vi "ADIS16448 Loop.vi"(8 "error in":errorcluster) -> ()   [LabVIEW 2019]
uses:
  Typedef/ADIS16448 Device Reference.ctl
  Typedef/ADIS16448 Hardware Configuration.ctl
  <vilib>/Rock Robotics/WPI/SPI/WPI_SPIMode.ctl
  <vilib>/Rock Robotics/SystemInterfaces/DIO/FPGA_DIOChannel.ctl
  <vilib>/Rock Robotics/SystemInterfaces/spilib/spi_bus.ctl
  Typedef/ADIS16448 Status.ctl
  Typedef/ADIS16448 Data.ctl
  Typedef/ADIS16448 Process.ctl
  Typedef/ADIS16448 Command Type.ctl
  <vilib>/Rock Robotics/SystemInterfaces/CounterEncoderSourceConvertion/FPGA_CounterEncoderSourceConvertionLVSourceType.ctl
  <vilib>/Rock Robotics/SystemInterfaces/DIO/FPGA_DIODigitalSourceChannel.ctl
  <vilib>/Rock Robotics/SystemInterfaces/AnalogTrigger/FPGA_AnalogTriggerIndex.ctl
  <vilib>/Rock Robotics/SystemInterfaces/AnalogTrigger/FPGA_AnalogTriggerOutType.ctl
  <vilib>/Rock Robotics/WPI/SPI/WPI_SPIDevRef.ctl
  Typedef/ADIS16448 Register.ctl
  <vilib>/Rock Robotics/WPI/Counter/WPI_CounterDigitalInputToDigitalSource.vi
  <vilib>/ptbypt/NI_PtbyPt.lvlib
panel:
  in  "Calibration Time":i32
  in  "element":T1
  in  "ADIS16448DevRef":T2={"DevStatus"={"status"=FALSE, "code"=0, "source"=""}, "Hardware Config"={"SPI Clock Rate (Hz)"=1000000.0, "IMU SPI Mode (3)"=enum."Mode 3 (Clk Idle High,Sample on Trailing)", "IMU Reset Pin"=enum."SPI Port CS2", "IMU SPI Bus"=enum."SPI On-Board, CS0", "IMU Data Ready Pin"=enum."SPI Port CS1", "Stall Config"={"Pow2BytesPerRead"=255, "StallTicks"=640, "CsToSclkTicks"=5}, "IMU Status LED Pin"=enum."DIO MXP 9"}, "Calibration Complete"=refnum, "Status FIFO"=refnum, "Last Value Reference"=refnum, "Sychronous Process VI"=refnum, "Cmd FIFO"=refnum, "Source"={"DevStatus"={"status"=FALSE, "code"=0, "source"=""}, "AnalogTriggerMode?"=FALSE, "DigitalMode"={"DIO Channel"=enum."Disabled"}, "AnalogTriggerMode"={"AnalogTriggerIndex"=enum."Trig 0", "OutputType"=enum."InWindow"}}, "Data FIFO"=refnum, "IMU Status LED Pin"=enum."DIO MXP 9", "Calibration Time"=5}
  in  "Main Name":string
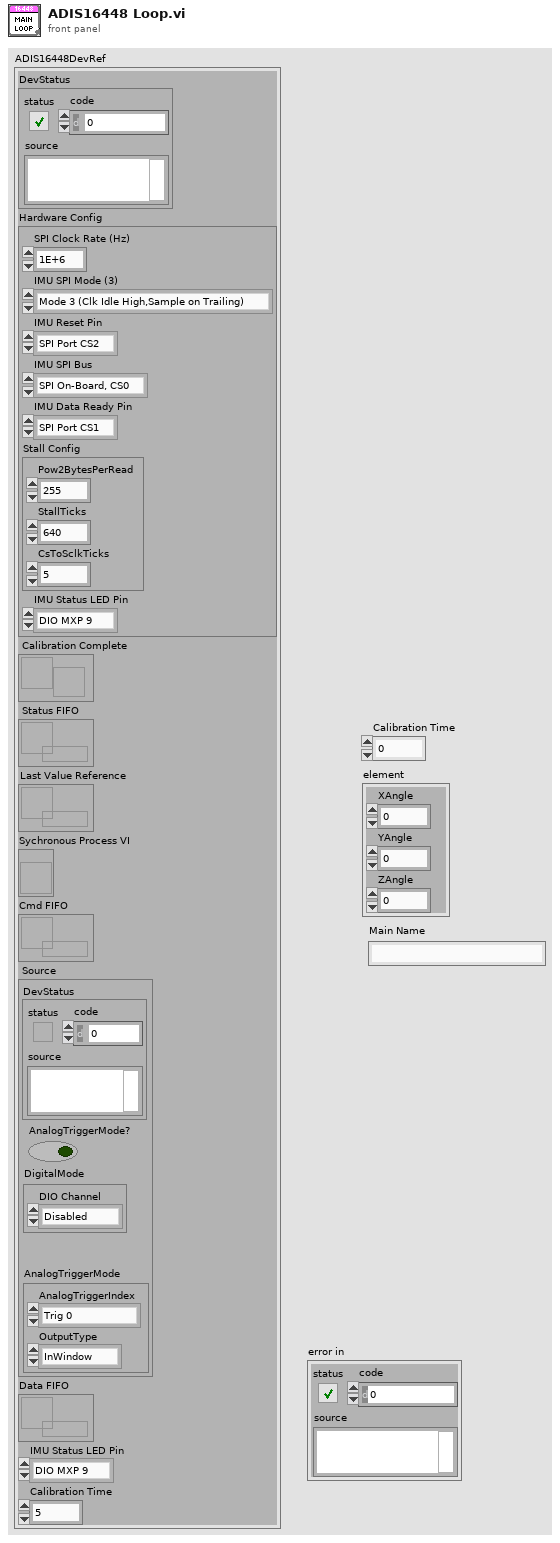
[diagram p1: front panel]
types:
  T1 = typedef "ADIS16448 Data.ctl" = cluster{"XAngle":dbl, "YAngle":dbl, "ZAngle":dbl}
  T2 = typedef "ADIS16448 Device Reference.ctl" = cluster{"DevStatus":errorcluster, "Hardware Config":T3, "Calibration Complete":refnum<notifier>, "Status FIFO":refnum<k33>, "Last Value Reference":refnum<data-value>, "Sychronous Process VI":T7, "Cmd FIFO":refnum<k33>, "Source":T8, "Data FIFO":refnum<k33>, "IMU Status LED Pin":T5, "Calibration Time":u32}
  T3 = typedef "ADIS16448 Hardware Configuration.ctl" = cluster{"SPI Clock Rate (Hz)":dbl, "IMU SPI Mode (3)":T4, "IMU Reset Pin":T5, "IMU SPI Bus":T6, "IMU Data Ready Pin":T5, "Stall Config":cluster{"Pow2BytesPerRead":u8, "StallTicks":u16, "CsToSclkTicks":u8}, "IMU Status LED Pin":T5}
  T4 = typedef "WPI_SPIMode.ctl" = enum16{"Mode 0 (Clk Idle Low,Sample on Leading)", "Mode 1 (Clk Idle Low,Sample on Trailing)", "Mode 2 (Clk Idle High,Sample on Leading)", "Mode 3 (Clk Idle High,Sample on Trailing)"}
  T5 = typedef "FPGA_DIOChannel.ctl" = enum8{"DIO 0", "DIO 1", "DIO 2", "DIO 3", "DIO 4", "DIO 5", "DIO 6", "DIO 7", "DIO 8", "DIO 9", "DIO MXP 0", "DIO MXP 1", "DIO MXP 2", "DIO MXP 3", "DIO MXP 4", "DIO MXP 5", "DIO MXP 6", "DIO MXP 7", "DIO MXP 8", "DIO MXP 9", "DIO MXP 10", "DIO MXP 11", "DIO MXP 12", "DIO MXP 13", "DIO MXP 14", "DIO MXP 15", "SPI Port CS1", "SPI Port CS2", "SPI Port CS3", "SPI Port MISO", "SPI Port MOSI", "Invalid"}
  T6 = typedef "spi_bus.ctl" = enum16{"SPI On-Board, CS0", "SPI On-Board, CS1", "SPI On-Board, CS2", "SPI On-Board, CS3", "SPI MXP", "Invalid"}
  T7 = typedef "ADIS16448 Process.ctl" = refnum<vi>
  T8 = typedef "FPGA_CounterEncoderSourceConvertionLVSourceType.ctl" = cluster{"DevStatus":errorcluster, "AnalogTriggerMode?":bool, "DigitalMode":cluster{"DIO Channel":T9}, "AnalogTriggerMode":cluster{"AnalogTriggerIndex":T10, "OutputType":T11}}
  T9 = typedef "FPGA_DIODigitalSourceChannel.ctl" = enum8{"DIO 0", "DIO 1", "DIO 2", "DIO 3", "DIO 4", "DIO 5", "DIO 6", "DIO 7", "DIO 8", "DIO 9", "DIO MXP 0", "DIO MXP 1", "DIO MXP 2", "DIO MXP 3", "DIO MXP 4", "DIO MXP 5", "DIO MXP 6", "DIO MXP 7", "DIO MXP 8", "DIO MXP 9", "DIO MXP 10", "DIO MXP 11", "DIO MXP 12", "DIO MXP 13", "DIO MXP 14", "DIO MXP 15", "SPI Port CS1", "SPI Port CS2", "SPI Port CS3", "SPI Port MISO", "SPI Port MOSI", "Disabled"}
  T10 = typedef "FPGA_AnalogTriggerIndex.ctl" = enum8{"Trig 0", "Trig 1", "Trig 2", "Trig 3", "Trig 4", "Trig 5", "Trig 6", "Trig 7", "Invalid"}
  T11 = typedef "FPGA_AnalogTriggerOutType.ctl" = enum16{"InWindow", "TriggerState", "Rising", "Falling"}
  T12 = typedef "WPI_SPIDevRef.ctl" = cluster{"DevStatus":errorcluster, "Handle":i32, "SPI Bus":T6}
  T13 = cluster{"SPIDevRef":T12, "Data Counter":u16, "Reset":bool, "Digital Source":T8, "Bytes Per Sample":u32, "Data":dbl[], "ADIS16448DevRef":T2, "TimeStampPrev":u32, "Sensor to Robot Rotation":dbl[][], "AutoSPI Active?":bool, "Offsets":dbl[], "Offset Counter":i32, "Data Header":u8[], "Zero Byte Count":u8, "Running Offset":dbl[]}
  T14 = typedef "ADIS16448 Status.ctl" = cluster{"Calibrated?":bool, "IMU Detected?":bool}
  T15 = typedef "ADIS16448 Register.ctl" = u8
  T16 = typedef "ADIS16448 Command Type.ctl" = cluster{"Command":enum16{"None", "Reset", "Rewrite Config", "Start Recal", "Recalibrate", "Recal Complete", "Exit Auto SPI", "Start Auto SPI", "Configure Cal"}, "Data":u32}
  T17 = typedef "WPI_DigitalOutputDevRef.ctl" = cluster{"DIO Channel":T5, "DevStatus":errorcluster}
  T18 = typedef "WPI_DigitalInputDevRef.ctl" = cluster{"DevStatus":errorcluster, "DIO Channel":T5}
  T19 = cluster{"Pow2BytesPerRead":u8, "StallTicks":u16, "CsToSclkTicks":u8}
  T20 = enum16{"None", "Reset", "Rewrite Config", "Start Recal", "Recalibrate", "Recal Complete", "Exit Auto SPI", "Start Auto SPI", "Configure Cal"}
  T21 = enum32{"Bad", "Idle", "Run top level", "Running"}
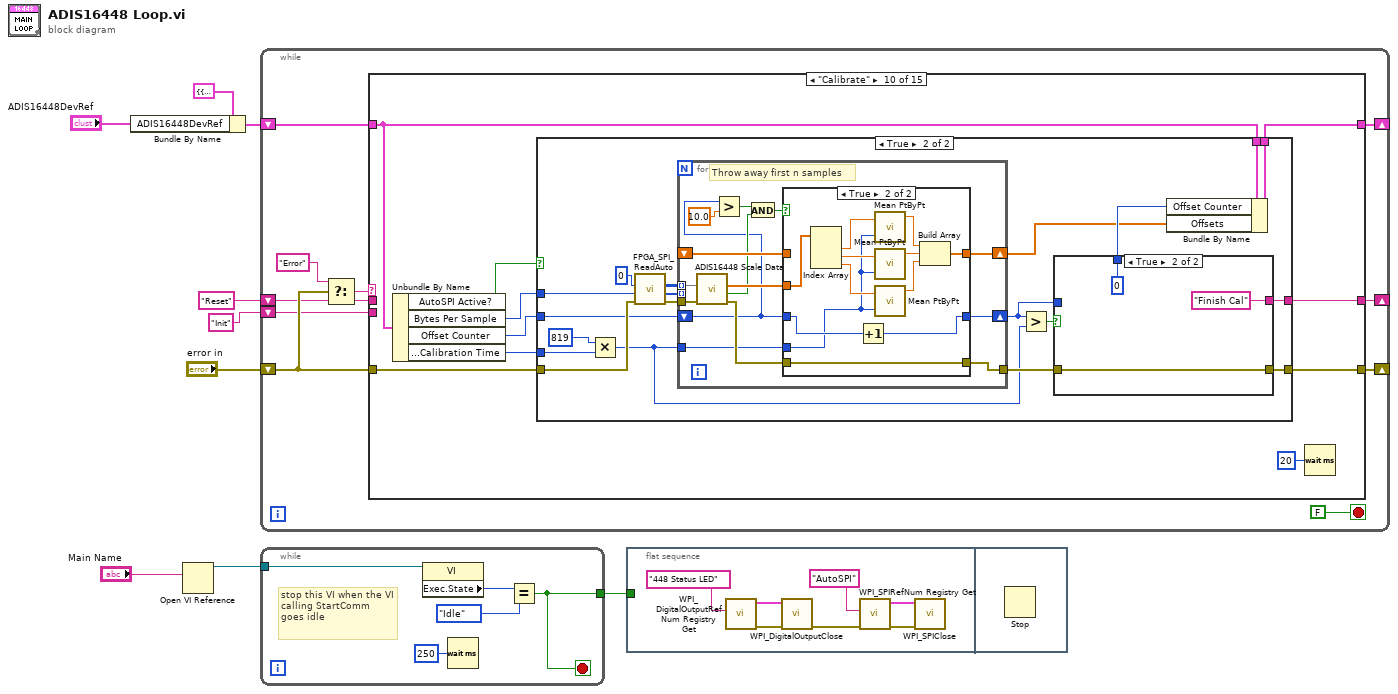
[diagram p0: block diagram]
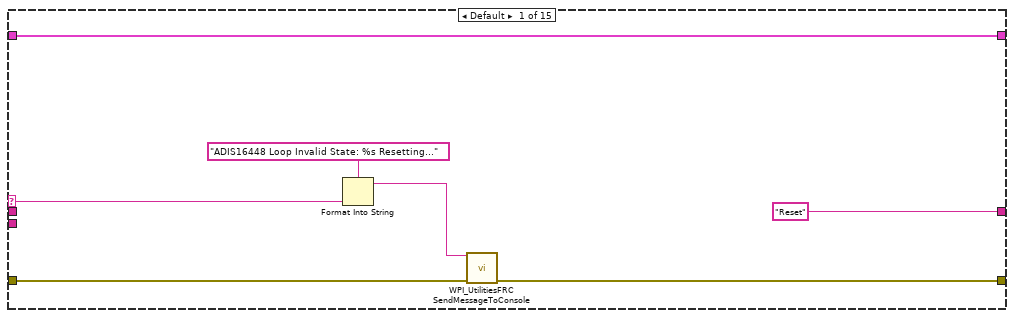
[diagram p2: hidden frame]
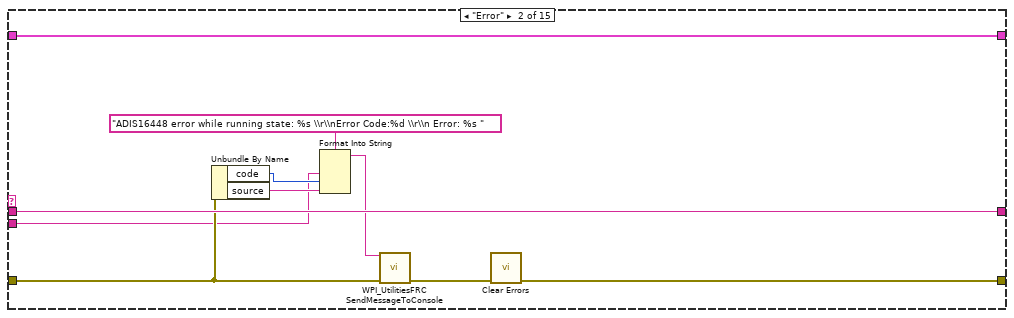
[diagram p3: hidden frame]
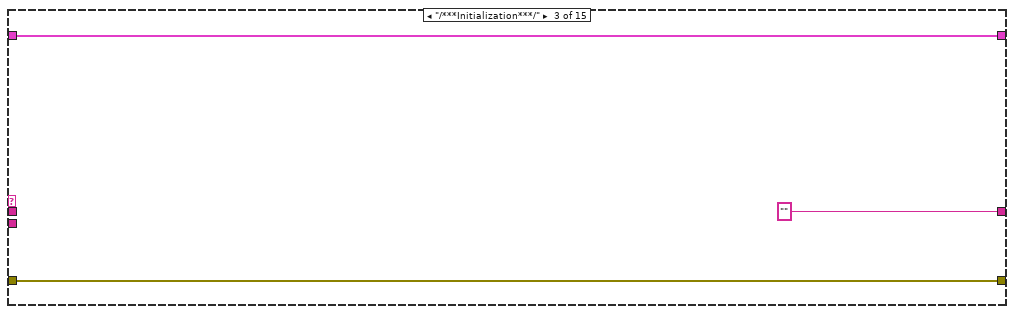
[diagram p4: hidden frame]
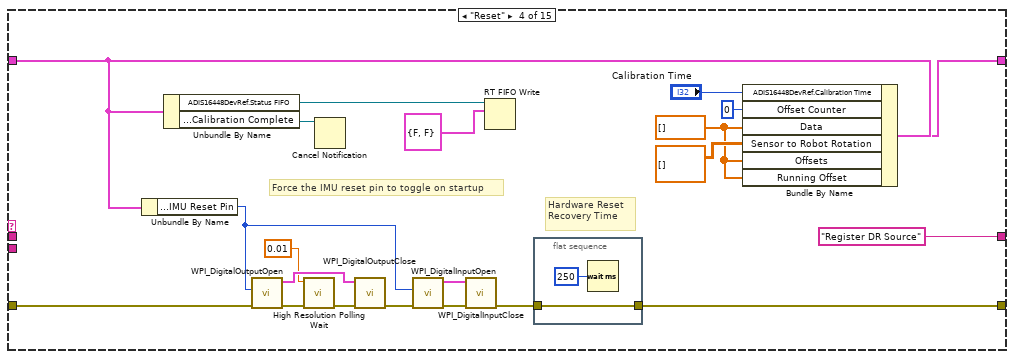
[diagram p5: hidden frame]
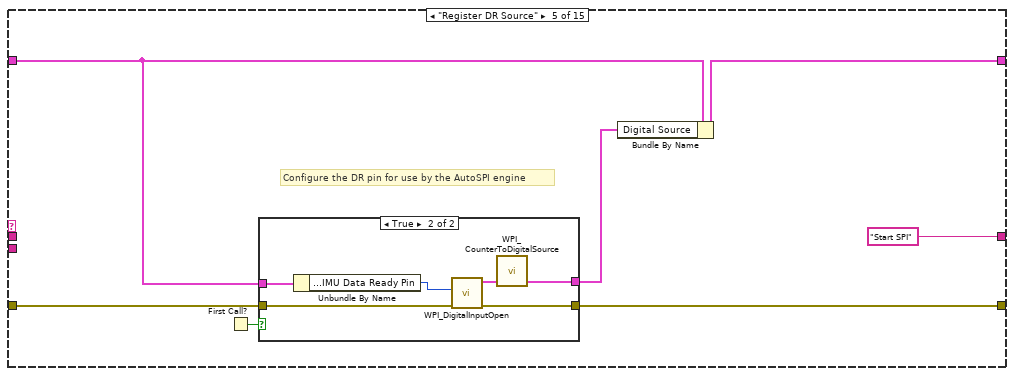
[diagram p6: hidden frame]
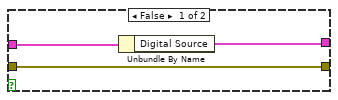
[diagram p7: hidden frame]
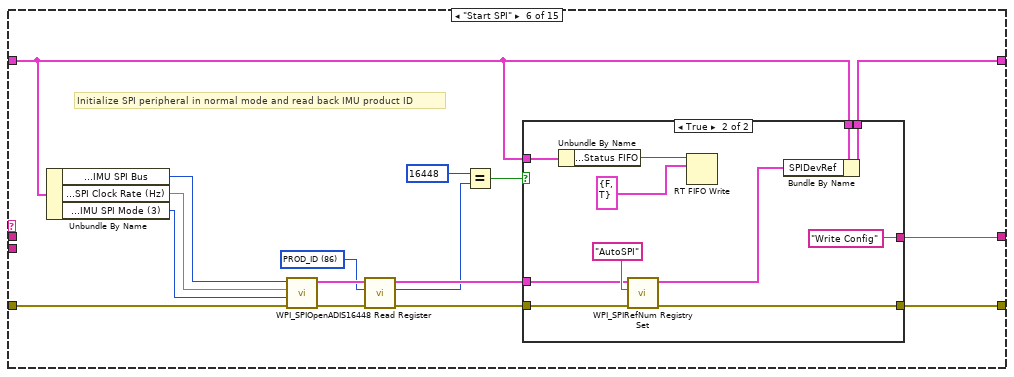
[diagram p8: hidden frame]
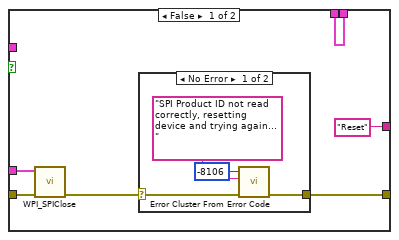
[diagram p9: hidden frame]
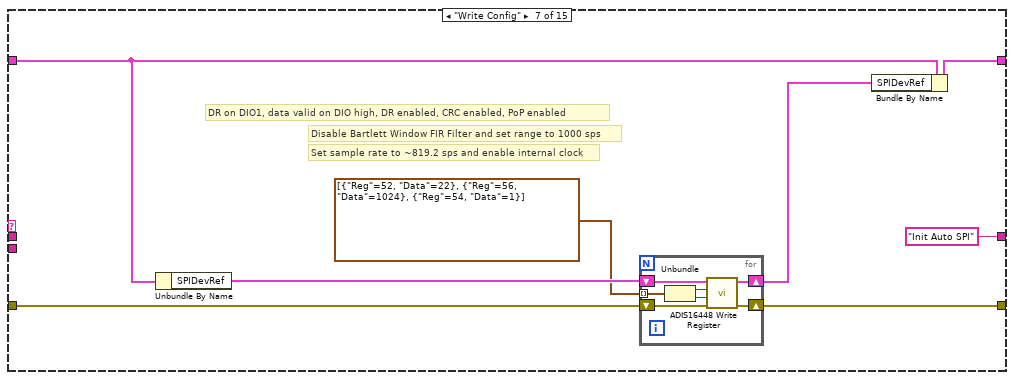
[diagram p11: hidden frame]
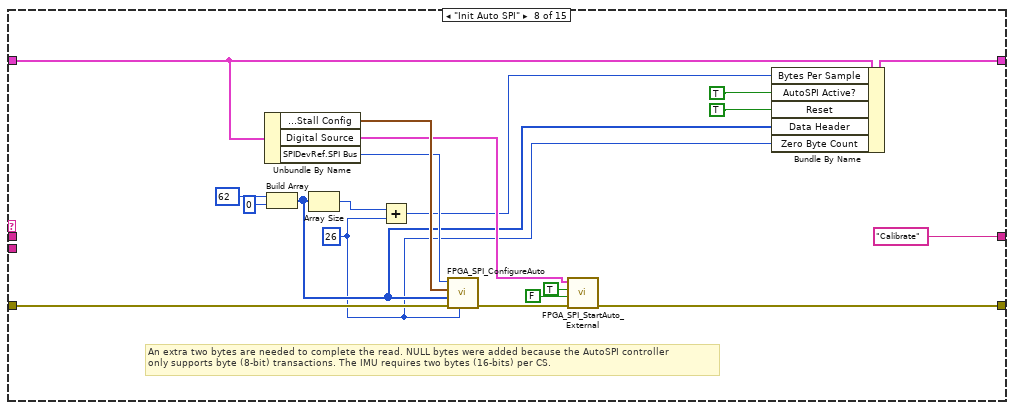
[diagram p12: hidden frame]
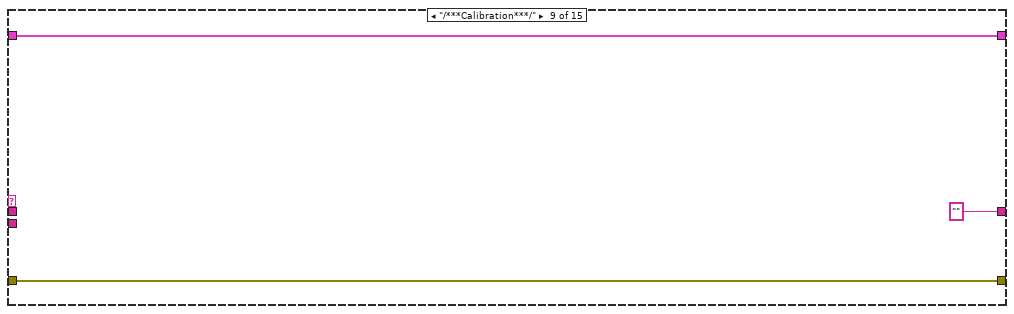
[diagram p13: hidden frame]
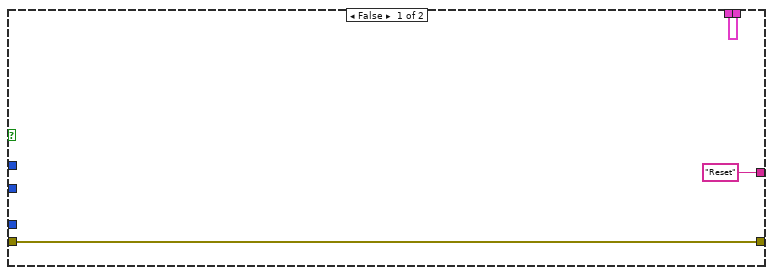
[diagram p14: hidden frame]
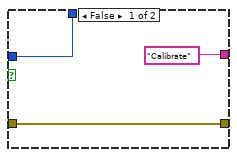
[diagram p15: hidden frame]
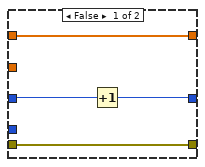
[diagram p16: hidden frame]
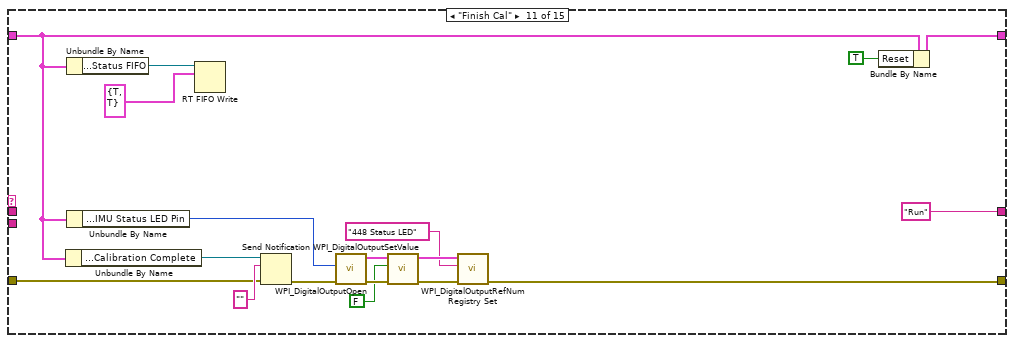
[diagram p17: hidden frame]
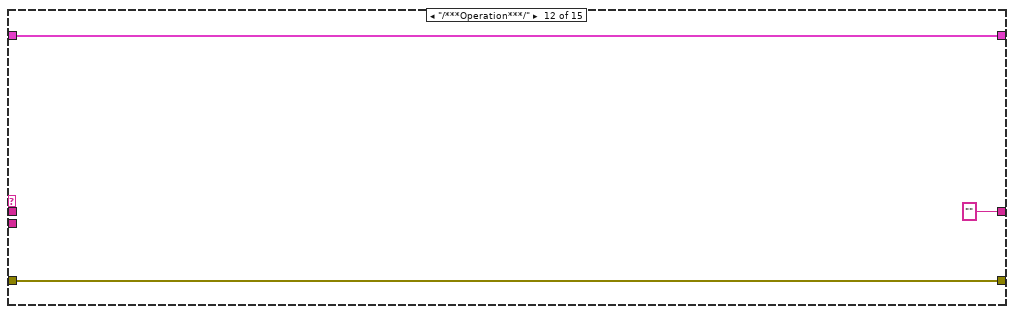
[diagram p18: hidden frame]
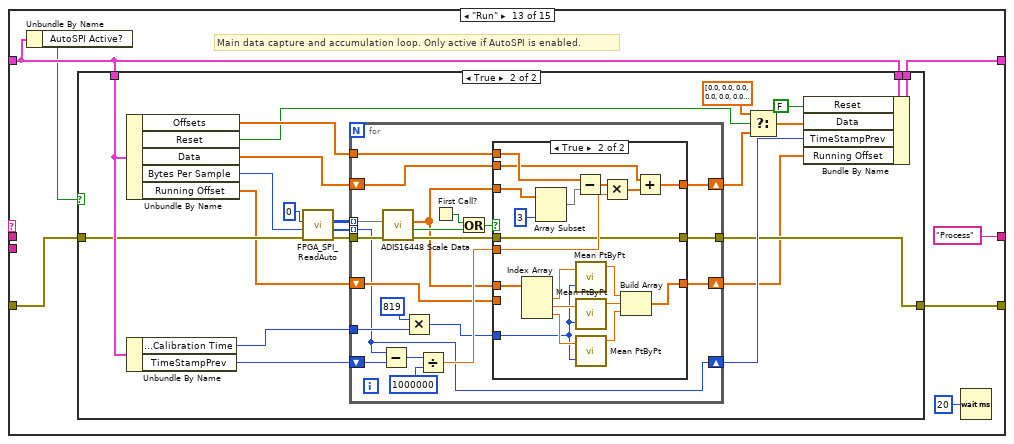
[diagram p19: hidden frame]
diagram:
  n1 = Bundle By Name(cluster=T13 {"SPIDevRef"={"DevStatus"={"status"=FALSE, "code"=0, "source"=""}, "Handle"=0, "SPI Bus"=enum."SPI On-Board, CS0"}, "Data Counter"=0, "Reset"=FALSE, "Digital Source"={"DevStatus"={"status"=FALSE, "code"=0, "source"=""}, "AnalogTriggerMode?"=FALSE, "DigitalMode"={"DIO Channel"=enum."DIO 1"}, "AnalogTriggerMode"={"AnalogTriggerIndex"=enum."Trig 0", "OutputType"=enum."InWindow"}}, "Bytes Per Sample"=0, "Data"=[0.0, 0.0, 0.0, 0.0, 0.0, 0.0, 0.0, 0.0], "ADIS16448DevRef"={"DevStatus"={"status"=FALSE, "code"=0, "source"=""}, "Hardware Config"={"SPI Clock Rate (Hz)"=1000000.0, "IMU SPI Mode (3)"=enum."Mode 3 (Clk Idle High,Sample on Trailing)", "IMU Reset Pin"=enum."SPI Port CS2", "IMU SPI Bus"=enum."SPI On-Board, CS0", "IMU Data Ready Pin"=enum."SPI Port CS1", "Stall Config"={"Pow2BytesPerRead"=255, "StallTicks"=640, "CsToSclkTicks"=5}, "IMU Status LED Pin"=enum."DIO MXP 9"}, "Calibration Complete"=refnum, "Status FIFO"=refnum, "Last Value Reference"=refnum, "Sychronous Process VI"=refnum, "Cmd FIFO"=refnum, "Source"={"DevStatus"={"status"=FALSE, "code"=0, "source"=""}, "AnalogTriggerMode?"=FALSE, "DigitalMode"={"DIO Channel"=enum."Disabled"}, "AnalogTriggerMode"={"AnalogTriggerIndex"=enum."Trig 0", "OutputType"=enum."InWindow"}}, "Data FIFO"=refnum, "IMU Status LED Pin"=enum."DIO MXP 9", "Calibration Time"=5}, "TimeStampPrev"=0, "Sensor to Robot Rotation"=[], "AutoSPI Active?"=TRUE, "Offsets"=[0.0, 0.0, 0.0, 0.0, 0.0, 0.0, 0.0, 0.0], "Offset Counter"=0, "Data Header"=[], "Zero Byte Count"=0, "Running Offset"=[0.0, 0.0, 0.0, 0.0, 0.0, 0.0, 0.0, 0.0]}, "ADIS16448DevRef"="ADIS16448DevRef") -> (w5:T13)
  n2 = Open VI Reference(vi path="Main Name") -> (vi reference=w8:refnum<vi>)  [unwired: 3 in, 3 out]
  n3 = while {
    shift-right: [w15] -> _
    shift-left: "Reset" -> [w12]
    shift-right: [w17] -> _
    shift-left: w5 -> [w18]
    shift-right: [w16] -> _
    shift-left: "error in" -> [w14]
    shift-left: "Init" -> [w10]
    stop <- FALSE stop-if-true
    n4 = Select(t="Error", s=w14, f=w12) -> (s? t:f=w13:string)
    n5 = case shown="\"Calibrate\"" w13 {
      selector: w13 -> [w25 _ _ _ _ _ _ _ _ _ _ _ _ _ _]
      tunnel: w18 -> [w26 w36 w39 w55 w64 w83 w119 w145 w153 w155 w231 w242 w244 w328 w338]
      tunnel: [w26 w36 w39 w54 w68 w88 w118 w144 w153 w160 w238 w242 w248 w328 w344] -> w17
      tunnel: w14 -> [w24 w32 w38 w48 w67 w94 w122 w149 w152 w162 w232 w241 w247 w326 w346]
      tunnel: [w23 w33 w38 w59 w65 w87 w121 w132 w152 w161 w224 w241 w246 w325 w345] -> w16
      tunnel: ["Reset" w35 "" "Register DR Source" "Start SPI" w89 "Init Auto SPI" "Calibrate" "" w156 "Run" "" "Process" "Run Cmds" w336] -> w15
      tunnel: w12 -> [_ w35 _ _ _ _ _ _ _ _ _ _ _ _ _]
      tunnel: w10 -> [_ w27 _ _ _ _ _ _ _ _ _ _ _ _ _]
      frame Default {
        n6 = Format Into String(format string="ADIS16448 Loop Invalid State: %s Resetting...", w25) -> (resulting string=w22:string)  [unwired: 2 in, 1 out]
        n7 = call <vilib>:"WPI_UtilitiesFRC SendMessageToConsole.vi"("Message"=w22, "error in (no error)"=w24) -> ("error out"=w23:errorcluster)  [unwired: 13 in]
      }
      frame "Error" {
        n8 = Unbundle By Name(w32) -> ("code"=w29:i32, "source"=w28:string)
        n9 = Format Into String(format string="ADIS16448 error while running state: %s \\r\\nError Code:%d \\r\\n Error: %s ", w27, w29, w28) -> (resulting string=w31:string)  [unwired: 2 in, 1 out]
        n10 = call <vilib>:"WPI_UtilitiesFRC SendMessageToConsole.vi"("Message"=w31, "error in (no error)"=w32) -> ("error out"=w34:errorcluster)  [unwired: 13 in]
        n11 = call <vilib>:"Clear Errors.vi"("error in (no error)"=w34) -> ("error out"=w33:errorcluster)  [unwired: 5 in, 1 out]
      }
      frame "/***Initialization***/" {
      }
      frame "Reset" {
        w40 = dbl[] [] ("Data")
        # "Hardware Reset Recovery Time"
        # "Force the IMU reset pin to toggle on startup"
        n12 = Unbundle By Name(w55) -> ("ADIS16448DevRef.Hardware Config.IMU Reset Pin"=w44:T5)
        n13 = Unbundle By Name(w55) -> ("ADIS16448DevRef.Status FIFO"=w57:refnum<k33>, "ADIS16448DevRef.Calibration Complete"=w58:refnum<notifier>)
        n14 = call <vilib>:"WPI_DigitalOutputOpen.vi"("error in (no error)"=w48, "DIO Channel"=w44) -> ("error out"=w46:errorcluster, "DigitalOutputDevRef"=w53:T17)  [unwired: 8 in]
        n15 = call <vilib>:"High Resolution Polling Wait.vi"("error in (no error)"=w46, "seconds to wait"=0.01) -> ("error out"=w47:errorcluster)  [unwired: 9 in]
        n16 = Cancel Notification(0:w58) -> ()  [unwired: 1 in, 3 out]
        n17 = call <vilib>:"WPI_DigitalOutputClose.vi"("error in (no error)"=w47, "DigitalOutputDevRef"=w53) -> ("error out"=w50:errorcluster)  [unwired: 9 in]
        n18 = call <vilib>:"WPI_DigitalInputOpen.vi"("error in (no error)"=w50, "DIO Channel"=w44) -> ("error out"=w51:errorcluster, "DigitalInputDevRef"=w52:T18)  [unwired: 8 in]
        n19 = call <vilib>:"WPI_DigitalInputClose.vi"("error in (no error)"=w51, "DigitalInputDevRef"=w52) -> ("error out"=w49:errorcluster)  [unwired: 9 in]
        n20 = RT FIFO Write(0:w57, 1:T14 {"Calibrated?"=FALSE, "IMU Detected?"=FALSE} ("element")) -> ()  [unwired: 3 in, 4 out]
        n21 = flat-sequence {
          tunnel: [w62] -> w59
          tunnel: w49 -> [w62]
          frame #0 {
            n22 = Wait (ms)(milliseconds to wait=u32 250) -> ()  [unwired: 1 out]
          }
        }
        n23 = Bundle By Name(cluster=w55, "ADIS16448DevRef.Calibration Time"="Calibration Time", "Offset Counter"=0, "Data"=w40, "Sensor to Robot Rotation"=dbl[][] [], "Offsets"=w40, "Running Offset"=w40) -> (w54:T13)
      }
      frame "Register DR Source" {
        # "Configure the DR pin for use by the AutoSPI engine"
        n24 = First Call?() -> (First Call?: T/F=w63:bool)
        n25 = case shown="True" w63 {
          tunnel: w67 -> [w70 w78]
          tunnel: w64 -> [w72 w76]
          tunnel: [w71 w74] -> w66
          tunnel: [w70 w73] -> w65
          frame False {
            n26 = Unbundle By Name(w72) -> ("Digital Source"=w71:T8)
          }
          frame True {
            n27 = Unbundle By Name(w76) -> ("ADIS16448DevRef.Hardware Config.IMU Data Ready Pin"=w75:T5)
            n28 = call <vilib>:"WPI_DigitalInputOpen.vi"("error in (no error)"=w78, "DIO Channel"=w75) -> ("error out"=w73:errorcluster, "DigitalInputDevRef"=w77:T18)  [unwired: 8 in]
            n29 = call-poly <vilib>:"WPI_CounterToDigitalSource.vi"("DigitalInputDevRef"=w77) -> ("Digital Source"=w74:T8)  [unwired: 6 in]
          }
        }
        n30 = Bundle By Name(cluster=w64, "Digital Source"=w66) -> (w68:T13)
      }
      frame "Start SPI" {
        w82 = T15 86 items=["FLASH_CNT"=0, "Reserved 1"=2, "XGYRO_OUT"=4, "YGYRO_OUT"=6, "ZGYRO_OUT"=8, "XACCL_OUT"=10, "YACCL_OUT"=12, "ZACCL_OUT"=14, "XMAGN_OUT"=16, "YMAGN_OUT"=18, "ZMAGN_OUT"=20, "BARO_OUT"=22, "TEMP_OUT"=24, "XGYRO_OFF"=26, "YGYRO_OFF"=28, "ZGYRO_OFF"=30, "XACCL_OFF"=32, "YACCL_OFF"=34, "ZACCL_OFF"=36, "XMAGN_HIC"=38, "YMAGN_HIC"=40, "ZMAGN_HIC"=42, "XMAGN_SIC"=44, "YMAGN_SIC"=46, "ZMAGN_SIC"=48, "GPIO_CTRL"=50, "MSC_CTRL"=52, "SMPL_PRD"=54, "SENS_AVG"=56, "SEQ_CNT"=58, "DIAG_STAT"=60, "GLOB_CMD"=62, "ALM_MAG1"=64, "ALM_MAG2"=66, "ALM_SMPL1"=68, "ALM_SMPL2"=70, "ALM_CTRL"=72, "Reserved 2"=74, "Reserved 3"=76, "Reserved 4"=78, "Reserved 5"=80, "LOT_ID1"=82, "LOT_ID2"=84, "PROD_ID"=86, "SERIAL_NUM"=88] ("ADIS16448 Register")
        # "Initialize SPI peripheral in normal mode and read back IMU product ID"
        n31 = Unbundle By Name(w83) -> ("ADIS16448DevRef.Hardware Config.IMU SPI Bus"=w90:T6, "ADIS16448DevRef.Hardware Config.SPI Clock Rate (Hz)"=w91:dbl, "ADIS16448DevRef.Hardware Config.IMU SPI Mode (3)"=w92:T4)
        n32 = call <vilib>:"WPI_SPIOpen.vi"("error in"=w94, "Mode (3)"=w92, "Clock Rate (Hz)"=w91, "SPI Bus"=w90) -> ("error out"=w86:errorcluster, "SPIDevRef"=w85:T12)  [unwired: 6 in]
        n33 = call "ADIS16448 Read Register.vi"("error in (no error)"=w86, "ADIS16448 Register"=w82, "SPIDevRef in"=w85) -> ("error out"=w80:errorcluster, "Register Value"=w79:u16, "SPIDevRef out"=w81:T12)  [unwired: 6 in]
        n34 = Equal?(x=u16 16448 ("y"), y=w79) -> (x = y?=w93:bool)
        n35 = case shown="True" w93 {
          tunnel: ["Reset" "Write Config"] -> w89
          tunnel: w83 -> [w99 w115]
          tunnel: [w99 w114] -> w88
          tunnel: [w98 w109] -> w87
          tunnel: w80 -> [w97 w110]
          tunnel: w81 -> [w96 w111]
          tunnel: w83 -> [_ w106]
          frame False {
            n36 = call <vilib>:"WPI_SPIClose.vi"("error in (no error)"=w97, "SPIDevRef"=w96) -> ("error out"=w95:errorcluster)  [unwired: 9 in]
            n37 = case shown="No Error" w95 {
              selector: w95 -> [w103 w105]
              tunnel: [w104 w105] -> w98
              frame No Error {
                n38 = call <vilib>:"Error Cluster From Error Code.vi"("error in (no error)"=w103, "error message (\"\")"="SPI Product ID not read correctly, resetting device and trying again..." ("error message (\"\")"), "error code (0)"=-8106) -> ("error out"=w104:errorcluster)  [unwired: 6 in]
              }
              frame Error {
              }
            }
          }
          frame True {
            n39 = Unbundle By Name(w106) -> ("ADIS16448DevRef.Status FIFO"=w108:refnum<k33>)
            n40 = call <vilib>:"WPI_SPIRefNum Registry Set.vi"("error in (no error)"=w110, "refnum name"="AutoSPI", "SPIDevRef"=w111) -> ("error out"=w109:errorcluster, "SPIDevRef"=w113:T12)  [unwired: 7 in]
            n41 = RT FIFO Write(0:w108, 1:T14 {"Calibrated?"=FALSE, "IMU Detected?"=TRUE} ("element")) -> ()  [unwired: 3 in, 4 out]
            n42 = Bundle By Name(cluster=w115, "SPIDevRef"=w113) -> (w114:T13)
          }
        }
      }
      frame "Write Config" {
        # "DR on DIO1, data valid on DIO high, DR enabled, CRC enabled, PoP enabled"
        # "Set sample rate to ~819.2 sps and enable internal clock"
        # "Disable Bartlett Window FIR Filter and set range to 1000 sps"
        n43 = Unbundle By Name(w119) -> ("SPIDevRef"=w123:T12)
        n44 = for {
          tunnel: cluster{"Reg":T15, "Data":u16}[] [{"Reg"=52, "Data"=22}, {"Reg"=56, "Data"=1024}, {"Reg"=54, "Data"=1}] -> [w131] mode=indexing
          shift-right: [w127] -> w121
          shift-left: w122 -> [w126]
          shift-right: [w125] -> w117
          shift-left: w123 -> [w128]
          n45 = Unbundle(w131) -> ("Reg"=w130:T15, "Data"=w129:u16)
          n46 = call "ADIS16448 Write Register.vi"("error in (no error)"=w126, "Data"=w129, "Register"=w130, "SPIDevRef in"=w128) -> ("error out"=w127:errorcluster, "SPIDevRef out"=w125:T12)  [unwired: 6 in]
        }
        n47 = Bundle By Name(cluster=w119, "SPIDevRef"=w117) -> (w118:T13)
      }
      frame "Init Auto SPI" {
        w133 = u8 26 ("dimension size")
        # "An extra two bytes are needed to complete the read. NULL bytes were added because the AutoSPI controller \nonly supports byte (8-bit) transactions. The IMU requires two bytes (16-bits) per CS."
        n48 = Unbundle By Name(w145) -> ("ADIS16448DevRef.Hardware Config.Stall Config"=w143:T19, "Digital Source"=w141:T8, "SPIDevRef.SPI Bus"=w140:T6)
        n49 = Build Array(u8 62 ("hi"), u8 0 ("element")) -> (w134:u8[])
        n50 = Array Size(array=w134) -> (size(s)=w138:i32)
        n51 = Add(x=w138, y=w133) -> (x+y=w135:i32)
        n52 = call <vilib>:"FPGA_SPI_ConfigureAuto.vi"("SPI Auto Zero Byte Count"=w133, "error in"=w149, "SPI Auto TX Byte Array"=w134, "Stall Config"=w143, "SPI Bus"=w140) -> ("error out"=w148:errorcluster)  [unwired: 6 in]
        n53 = call <vilib>:"FPGA_SPI_StartAuto_External.vi"("error in (no error)"=w148, "Falling Edge"=FALSE, "Rising Edge"=TRUE, "Source"=w141) -> ("error out"=w132:errorcluster)  [unwired: 7 in]
        n54 = Bundle By Name(cluster=w145, "Bytes Per Sample"=w135, "AutoSPI Active?"=TRUE, "Reset"=TRUE, "Data Header"=w134, "Zero Byte Count"=w133) -> (w144:T13)
      }
      frame "/***Calibration***/" {
      }
      frame "Calibrate" {
        n55 = Unbundle By Name(w155) -> ("AutoSPI Active?"=w163:bool, "Bytes Per Sample"=w159:u32, "Offset Counter"=w158:i32, "ADIS16448DevRef.Calibration Time"=w157:u32)
        n56 = case shown="True" w163 {
          tunnel: [w166 w185] -> w160
          tunnel: w162 -> [w165 w180]
          tunnel: [w165 w170] -> w161
          tunnel: w155 -> [w166 w181]
          tunnel: w159 -> [_ w178]
          tunnel: w158 -> [_ w175]
          tunnel: w157 -> [_ w176]
          tunnel: ["Reset" w171] -> w156
          frame False {
          }
          frame True {
            n57 = Multiply(x=819, y=w176) -> (x*y=w167:u32)
            n58 = call <vilib>:"FPGA_SPI_ReadAuto.vi"("error in (no error)"=w180, "Bytes per Sample"=w178, "Samples to Read"=u32 0) -> ("error out"=w179:errorcluster, "Timestamps"=w182:u32[], "Data"=w183:u8[][])  [unwired: 6 in]
            n59 = for {
              tunnel: w183 -> [w205] mode=indexing
              tunnel: w182 -> [_] mode=indexing
              tunnel: w179 -> [w204]
              tunnel: [w201] -> w169
              shift-right: [w202] -> w173
              shift-left: w175 -> [w193]
              shift-right: [w199] -> w168
              shift-left: _ -> [w198]
              tunnel: w167 -> [w197]
              # "Throw away first n samples"
              n60 = call "ADIS16448 Scale Data.vi"("error in (no error)"=w204, "New Data In"=w205) -> ("error out"=w200:errorcluster, "Data Good?"=w195:bool, "Data Out"=w203:dbl[])  [unwired: 7 in]
              n61 = Greater?(x=w193, y=10.0) -> (0:w192:bool)
              n62 = And(x=w192, y=w195) -> (x .and. y?=w194:bool)
              n63 = case shown="True" w194 {
                tunnel: w203 -> [_ w215]
                tunnel: w193 -> [w207 w212]
                tunnel: [w206 w211] -> w202
                tunnel: [w209 w213] -> w201
                tunnel: w200 -> [w209 w213]
                tunnel: [w208 w214] -> w199
                tunnel: w198 -> [w208 _]
                tunnel: w197 -> [_ w210]
                frame False {
                  n64 = Increment(x=w207) -> (x+1=w206:i32)
                }
                frame True {
                  n65 = Index Array(array=w215) -> (element #1=w216:dbl, element #2=w217:dbl, element #3=w218:dbl)  [unwired: 3 in]
                  n66 = Increment(x=w212) -> (x+1=w211:i32)
                  n67 = call <vilib>:"Mean PtByPt.vi"("x"=w216, "sample length"=w210) -> ("mean"=w219:dbl)  [unwired: 2 in, 1 out]
                  n68 = call <vilib>:"Mean PtByPt.vi"("x"=w217, "sample length"=w210) -> ("mean"=w220:dbl)  [unwired: 2 in, 1 out]
                  n69 = call <vilib>:"Mean PtByPt.vi"("x"=w218, "sample length"=w210) -> ("mean"=w221:dbl)  [unwired: 2 in, 1 out]
                  n70 = Build Array(w219, w220, w221) -> (w214:dbl[])
                }
              }
            }
            n71 = Greater?(x=w173, y=w167) -> (0:w174:bool)
            n72 = case shown="True" w174 {
              tunnel: w173 -> [w188 _]
              tunnel: [w188 u32 0 ("Offset Counter")] -> w172
              tunnel: ["Calibrate" "Finish Cal"] -> w171
              tunnel: [w186 w189] -> w170
              tunnel: w169 -> [w186 w189]
              frame False {
              }
              frame True {
              }
            }
            n73 = Bundle By Name(cluster=w181, "Offset Counter"=w172, "Offsets"=w168) -> (w185:T13)
          }
        }
        n74 = Wait (ms)(milliseconds to wait=u32 20) -> ()  [unwired: 1 out]
      }
      frame "Finish Cal" {
        n75 = Unbundle By Name(w231) -> ("ADIS16448DevRef.Calibration Complete"=w236:refnum<notifier>)
        n76 = Unbundle By Name(w231) -> ("ADIS16448DevRef.Status FIFO"=w234:refnum<k33>)
        n77 = Unbundle By Name(w231) -> ("ADIS16448DevRef.Hardware Config.IMU Status LED Pin"=w222:T5)
        n78 = RT FIFO Write(0:w234, 1:T14 {"Calibrated?"=TRUE, "IMU Detected?"=TRUE} ("element")) -> ()  [unwired: 3 in, 4 out]
        n79 = Send Notification(notification="", notifier=w236, error in (no error)=w232) -> (error out=w225:errorcluster)  [unwired: 1 out]
        n80 = call <vilib>:"WPI_DigitalOutputOpen.vi"("error in (no error)"=w225, "DIO Channel"=w222) -> ("error out"=w230:errorcluster, "DigitalOutputDevRef"=w229:T17)  [unwired: 8 in]
        n81 = call <vilib>:"WPI_DigitalOutputSetValue.vi"("error in (no error)"=w230, "Value"=FALSE, "DigitalOutputDevRef"=w229) -> ("error out"=w228:errorcluster, "DigitalOutputDevRef"=w227:T17)  [unwired: 7 in]
        n82 = call <vilib>:"WPI_DigitalOutputRefNum Registry Set.vi"("error in (no error)"=w228, "refnum name"="448 Status LED", "DigitalOutputDevRef"=w227) -> ("error out"=w224:errorcluster)  [unwired: 7 in, 1 out]
        n83 = Bundle By Name(cluster=w231, "Reset"=TRUE ("First Run")) -> (w238:T13)
      }
      frame "/***Operation***/" {
      }
      frame "Run" {
        # "Main data capture and accumulation loop. Only active if AutoSPI is enabled."
        n84 = Unbundle By Name(w244) -> ("AutoSPI Active?"=w243:bool)
        n85 = case shown="True" w243 {
          tunnel: [w251 w273] -> w248
          tunnel: w247 -> [w250 w259]
          tunnel: [w250 w256] -> w246
          tunnel: w244 -> [w251 w263]
          tunnel: w244 -> [_ w260]
          frame False {
          }
          frame True {
            n86 = Unbundle By Name(w260) -> ("Offsets"=w257:dbl[], "Reset"=w255:bool, "Data"=w267:dbl[], "Bytes Per Sample"=w271:u32, "Running Offset"=w253:dbl[])
            n87 = Unbundle By Name(w260) -> ("ADIS16448DevRef.Calibration Time"=w254:u32, "TimeStampPrev"=w262:u32)
            n88 = call <vilib>:"FPGA_SPI_ReadAuto.vi"("error in (no error)"=w259, "Bytes per Sample"=w271, "Samples to Read"=u32 0) -> ("error out"=w258:errorcluster, "Timestamps"=w268:u32[], "Data"=w269:u8[][])  [unwired: 6 in]
            n89 = for {
              tunnel: w269 -> [w293] mode=indexing
              tunnel: w268 -> [w274] mode=indexing
              shift-right: [w287] -> w266
              shift-left: w267 -> [w286]
              shift-right: [w274] -> w261
              shift-left: w262 -> [w294]
              tunnel: w258 -> [w292]
              tunnel: w257 -> [w291]
              tunnel: [w284] -> w256
              tunnel: w254 -> [w279]
              shift-right: [w275] -> w252
              shift-left: w253 -> [w276]
              n90 = Subtract(x=w274, y=w294) -> (x-y=w290:u32)
              n91 = call "ADIS16448 Scale Data.vi"("error in (no error)"=w292, "New Data In"=w293) -> ("error out"=w285:errorcluster, "Data Good?"=w282:bool, "Data Out"=w280:dbl[])  [unwired: 7 in]
              n92 = Multiply(x=819, y=w279) -> (x*y=w277:u32)
              n93 = Divide(x=w290, y=u32 1000000) -> (x/y=w288:dbl)
              n94 = First Call?() -> (First Call?: T/F=w281:bool)
              n95 = Or(x=w281, y=w282) -> (x .or. y?=w283:bool)
              n96 = case shown="True" w283 {
                tunnel: w280 -> [_ w315]
                tunnel: w291 -> [_ w313]
                tunnel: w288 -> [_ w311]
                tunnel: [w297 w310] -> w287
                tunnel: w286 -> [w297 w308]
                tunnel: w285 -> [w296 w307]
                tunnel: [w296 w307] -> w284
                tunnel: w280 -> [_ w300]
                tunnel: w277 -> [_ w299]
                tunnel: w276 -> [w295 _]
                tunnel: [w295 w298] -> w275
                frame False {
                }
                frame True {
                  n97 = Index Array(array=w300) -> (element #1=w301:dbl, element #2=w302:dbl, element #3=w303:dbl)  [unwired: 3 in]
                  n98 = Array Subset(array=w315, length=3) -> (w314:dbl[])  [unwired: 1 in]
                  n99 = Subtract(x=w313, y=w314) -> (x-y=w312:dbl[])
                  n100 = call <vilib>:"Mean PtByPt.vi"("x"=w301, "sample length"=w299) -> ("mean"=w304:dbl)  [unwired: 2 in, 1 out]
                  n101 = call <vilib>:"Mean PtByPt.vi"("x"=w302, "sample length"=w299) -> ("mean"=w305:dbl)  [unwired: 2 in, 1 out]
                  n102 = call <vilib>:"Mean PtByPt.vi"("x"=w303, "sample length"=w299) -> ("mean"=w306:dbl)  [unwired: 2 in, 1 out]
                  n103 = Multiply(x=w312, y=w311) -> (x*y=w309:dbl[])
                  n104 = Build Array(w304, w305, w306) -> (w298:dbl[])
                  n105 = Add(x=w308, y=w309) -> (x+y=w310:dbl[])
                }
              }
            }
            n106 = Select(t=dbl[] [0.0, 0.0, 0.0, 0.0, 0.0, 0.0, 0.0, 0.0] ("Angle and Vel"), s=w255, f=w266) -> (s? t:f=w264:dbl[])
            n107 = Bundle By Name(cluster=w263, "Reset"=FALSE ("First Run"), "Data"=w264, "TimeStampPrev"=w261, "Running Offset"=w252) -> (w273:T13)
          }
        }
        n108 = Wait (ms)(milliseconds to wait=u32 20) -> ()  [unwired: 1 out]
      }
      frame "Process" {
        n109 = Unbundle By Name(w328) -> ("ADIS16448DevRef.Sychronous Process VI"=w323:T7, "ADIS16448DevRef.Data FIFO"=w327:refnum<k33>, "Data"=w322:dbl[])
        n110 = Index Array(array=w322) -> (element #1=w321:dbl, element #2=w320:dbl, element #3=w319:dbl)  [unwired: 3 in]
        n111 = Bundle By Name(cluster="element", "XAngle"=w321, "YAngle"=w320, "ZAngle"=w319) -> (w317:T1)
        n112 = RT FIFO Write(0:w327, 1:w317) -> ()  [unwired: 3 in, 4 out]
        n113 = Not A Number/Path/Refnum?(number/path/refnum=w323) -> (NaN/Path/Refnum?=w324:bool)
        n114 = case shown="False" w324 {
          tunnel: w326 -> [w330 w335]
          tunnel: w317 -> [_ _]
          tunnel: [w334 w335] -> w325
          tunnel: w323 -> [w333 _]
          frame False {
            n115 = call-by-ref "?"(reference=w333, error in=w330, 8:"error in (no error)"=w330) -> (error out=w331:errorcluster, 0:"error out"=w332:errorcluster)  [unwired: 10 in, 1 out]
            n116 = Merge Errors(w331, w332) -> (w334:errorcluster)
          }
          frame True {
          }
        }
      }
      frame "Run Cmds" {
        n117 = Unbundle By Name(w338) -> ("ADIS16448DevRef.Cmd FIFO"=w347:refnum<k33>)
        n118 = Unbundle By Name(w338) -> ("ADIS16448DevRef.Status FIFO"=w342:refnum<k33>, "ADIS16448DevRef.Calibration Complete"=w343:refnum<notifier>)
        n119 = RT FIFO Read(0:w347, 1:T16 {"Command"=enum."None", "Data"=0} ("element")) -> (8:w341:refnum<k33>, 9:w340:T16)  [unwired: 2 in, 3 out]
        n120 = Unbundle(w340) -> ("Command"=w337:T20, "Data"=w339:u32)
        n121 = case shown="\"Exit Auto SPI\"" w337 {
          tunnel: w338 -> [w350 w356 w365 w376 w385 w403 w449 w466 w473]
          tunnel: w346 -> [w351 w355 w363 w373 w390 w419 w459 w469 w474]
          tunnel: [w351 w355 w362 w373 w390 w406 w450 w469 w474] -> w345
          tunnel: [w350 w354 w365 w377 w384 w402 w449 w466 w472] -> w344
          tunnel: w343 -> [_ _ _ _ w389 _ _ _ _]
          tunnel: w342 -> [_ _ _ _ w387 w394 _ w467 _]
          tunnel: w341 -> [_ _ w360 w380 _ w417 w461 w463 _]
          tunnel: w339 -> [_ _ _ _ _ _ _ _ w470]
          tunnel: w338 -> [_ _ w359 w378 _ w400 w448 _ _]
          tunnel: ["Run" "Run" "Run" "Run" "Run" w391 "Run" "Run" "Run"] -> w336
          frame "None", Default {
          }
          frame "Reset" {
            n122 = Bundle By Name(cluster=w356, "Reset"=TRUE ("First Run")) -> (w354:T13)
          }
          frame "Rewrite Config" {
            n123 = Unbundle By Name(w359) -> ("SPIDevRef"=w358:T12)
            n124 = RT FIFO Write(0:w360, 1:T16 {"Command"=enum."Start Auto SPI", "Data"=0} ("element")) -> ()  [unwired: 3 in, 4 out]
            n125 = for {
              tunnel: cluster{"Reg":T15, "Data":u16}[] [{"Reg"=52, "Data"=22}, {"Reg"=56, "Data"=1026}, {"Reg"=54, "Data"=1}] -> [w372] mode=indexing
              shift-right: [w368] -> w362
              shift-left: w363 -> [w367]
              shift-right: [w366] -> _
              shift-left: w358 -> [w369]
              n126 = Unbundle(w372) -> ("Reg"=w371:T15, "Data"=w370:u16)
              n127 = call "ADIS16448 Write Register.vi"("error in (no error)"=w367, "Data"=w370, "Register"=w371, "SPIDevRef in"=w369) -> ("error out"=w368:errorcluster, "SPIDevRef out"=w366:T12)  [unwired: 6 in]
            }
          }
          frame "Recalibrate" {
            n128 = Unbundle By Name(w378) -> ("Running Offset"=w375:dbl[])
            n129 = RT FIFO Write(0:w380, 1:T16 {"Command"=enum."Recal Complete", "Data"=0} ("element")) -> ()  [unwired: 3 in, 4 out]
            n130 = Bundle By Name(cluster=w376, "Offsets"=w375) -> (w377:T13)
          }
          frame "Recal Complete" {
            n131 = Send Notification(notification="", notifier=w389) -> ()  [unwired: 1 in, 2 out]
            n132 = RT FIFO Write(0:w387, 1:T14 {"Calibrated?"=TRUE, "IMU Detected?"=TRUE} ("element")) -> ()  [unwired: 3 in, 4 out]
            n133 = Bundle By Name(cluster=w385, "AutoSPI Active?"=TRUE, "Reset"=TRUE) -> (w384:T13)
          }
          frame "Exit Auto SPI" {
            w413 = T15 114 items=["Reserved1"=0, "DIAG_STAT"=2, "X_GYRO_LOW"=4, "X_GYRO_OUT"=6, "Y_GYRO_LOW"=8, "Y_GYRO_OUT"=10, "Z_GYRO_LOW"=12, "Z_GYRO_OUT"=14, "X_ACCL_LOW"=16, "X_ACCL_OUT"=18, "Y_ACCL_LOW"=20, "Y_ACCL_OUT"=22, "Z_ACCL_LOW"=24, "Z_ACCL_OUT"=26, "TEMP_OUT"=28, "TIME_STAMP"=30, "Reseved2"=32, "DATA_CNTR"=34, "X_DELTANG_LOW"=36, "X_DELTANG_OUT"=38, "Y_DELTANG_LOW"=40, "Y_DELTANG_OUT"=42, "Z_DELTANG_LOW"=44, "Z_DELTANG_OUT"=46, "X_DELTVEL_LOW"=48, "X_DELTVEL_OUT"=50, "Y_DELTVEL_LOW"=52, "Y_DELTVEL_OUT"=54, "Z_DELTVEL_LOW"=56, "Z_DELTVEL_OUT"=58, "Reserved3"=60, "Reserved4"=62, "XG_BIAS_LOW"=64, "XG_BIAS_HIGH"=66, "YG_BIAS_LOW"=68, "YG_BIAS_OUT"=70, "ZG_BIAS_LOW"=72, "ZG_BIAS_OUT"=74, "XA_BIAS_LOW"=76, "XA_BIAS_HIGH"=78, "YA_BIAS_LOW"=80, "YA_BIAS_OUT"=82, "ZA_BIAS_LOW"=84, "ZA_BIAS_OUT"=86, "Reserved5"=88, "Reserved6"=90, "FILT_CTRL"=92, "Reserved5"=94, "MSC_CTRL"=96, "UP_SCALE"=98, "DEC_RATE"=100, "NULL_CNFG"=102, "GLOB_CMD"=104, "Reserved6"=106, "FIRM_REV"=108, "FIRM_DM"=110, "FIRM_Y"=112, "PROD_ID"=114, "SERIAL_NUM"=116, "USER_SCR1"=118, "USER_SCR2"=120, "USER_SCR3"=122, "FLSHCNT_LOW"=124, "FLSHCNT_HIGH"=126] ("ADIS16448 Register")
            n134 = Unbundle By Name(w400) -> ("ADIS16448DevRef.Hardware Config.IMU SPI Bus"=w416:T6, "ADIS16448DevRef.Hardware Config.SPI Clock Rate (Hz)"=w415:dbl, "ADIS16448DevRef.Hardware Config.IMU SPI Mode (3)"=w414:T4, "SPIDevRef"=w395:T12)
            n135 = RT FIFO Write(0:w394, 1:T14 {"Calibrated?"=FALSE, "IMU Detected?"=FALSE} ("element")) -> (8:w392:refnum<k33>)  [unwired: 3 in, 3 out]
            n136 = RT FIFO Write(0:w417, 1:T16 {"Command"=enum."Rewrite Config", "Data"=0} ("element")) -> ()  [unwired: 3 in, 4 out]
            n137 = call <vilib>:"WPI_SPIClose.vi"("error in (no error)"=w419, "SPIDevRef"=w395) -> ("error out"=w404:errorcluster)  [unwired: 9 in]
            n138 = call <vilib>:"WPI_DigitalOutputRefNum Registry Get.vi"("error in (no error)"=w404, "refnum name"="448 Status LED") -> ("error out"=w398:errorcluster, "DigitalOutputDevRef"=w397:T17)  [unwired: 8 in]
            n139 = call <vilib>:"WPI_DigitalOutputSetValue.vi"("error in (no error)"=w398, "Value"=TRUE, "DigitalOutputDevRef"=w397) -> ("error out"=w399:errorcluster)  [unwired: 7 in, 1 out]
            n140 = call <vilib>:"WPI_SPIOpen.vi"("error in"=w399, "Mode (3)"=w414, "Clock Rate (Hz)"=w415, "SPI Bus"=w416) -> ("error out"=w412:errorcluster, "SPIDevRef"=w408:T12)  [unwired: 6 in]
            n141 = call "ADIS16448 Read Register.vi"("error in (no error)"=w412, "ADIS16448 Register"=w413, "SPIDevRef in"=w408) -> ("error out"=w409:errorcluster, "Register Value"=w407:u16, "SPIDevRef out"=w410:T12)  [unwired: 6 in]
            n142 = Equal?(x=u16 16448 ("y"), y=w407) -> (x = y?=w411:bool)
            n143 = case shown="True" w411 {
              tunnel: w410 -> [w422 w439]
              tunnel: w409 -> [w423 w438]
              tunnel: [w425 w437] -> w406
              tunnel: w403 -> [w424 w435]
              tunnel: [w424 w434] -> w402
              tunnel: w392 -> [_ w433]
              tunnel: ["Reset" "Run"] -> w391
              frame False {
                n144 = call <vilib>:"WPI_SPIClose.vi"("error in (no error)"=w423, "SPIDevRef"=w422) -> ("error out"=w421:errorcluster)  [unwired: 9 in]
                n145 = case shown="No Error" w421 {
                  selector: w421 -> [w427 w430]
                  tunnel: [w426 w430] -> w425
                  frame No Error {
                    n146 = call <vilib>:"Error Cluster From Error Code.vi"("error in (no error)"=w427, "error message (\"\")"="SPI port did not reset properly" ("error message (\"\")"), "error code (0)"=-8106) -> ("error out"=w426:errorcluster)  [unwired: 6 in]
                  }
                  frame Error {
                  }
                }
              }
              frame True {
                n147 = call <vilib>:"WPI_SPIRefNum Registry Set.vi"("error in (no error)"=w438, "refnum name"="AutoSPI", "SPIDevRef"=w439) -> ("error out"=w437:errorcluster, "SPIDevRef"=w440:T12)  [unwired: 7 in]
                n148 = RT FIFO Write(0:w433, 1:T14 {"Calibrated?"=FALSE, "IMU Detected?"=TRUE} ("element")) -> ()  [unwired: 3 in, 4 out]
                n149 = Bundle By Name(cluster=w435, "SPIDevRef"=w440, "AutoSPI Active?"=FALSE) -> (w434:T13)
              }
            }
          }
          frame "Start Auto SPI" {
            n150 = Unbundle By Name(w448) -> ("SPIDevRef"=w447:T12, "Digital Source"=w446:T8, "ADIS16448DevRef.Hardware Config.Stall Config"=w445:T19, "Data Header"=w444:u8[], "Zero Byte Count"=w443:u8)
            n151 = Unbundle By Name(w447) -> ("SPI Bus"=w460:T6)
            n152 = RT FIFO Write(0:w461, 1:T16 {"Command"=enum."Recal Complete", "Data"=0} ("element")) -> ()  [unwired: 3 in, 4 out]
            n153 = call <vilib>:"FPGA_SPI_ConfigureAuto.vi"("SPI Auto Zero Byte Count"=w443, "error in"=w459, "SPI Auto TX Byte Array"=w444, "Stall Config"=w445, "SPI Bus"=w460) -> ("error out"=w452:errorcluster)  [unwired: 6 in]
            n154 = call <vilib>:"FPGA_SPI_StartAuto_External.vi"("error in (no error)"=w452, "Falling Edge"=FALSE, "Rising Edge"=TRUE, "Source"=w446) -> ("error out"=w456:errorcluster)  [unwired: 7 in]
            n155 = call <vilib>:"WPI_DigitalOutputRefNum Registry Get.vi"("error in (no error)"=w456, "refnum name"="448 Status LED") -> ("error out"=w455:errorcluster, "DigitalOutputDevRef"=w454:T17)  [unwired: 8 in]
            n156 = call <vilib>:"WPI_DigitalOutputSetValue.vi"("error in (no error)"=w455, "Value"=FALSE, "DigitalOutputDevRef"=w454) -> ("error out"=w450:errorcluster)  [unwired: 7 in, 1 out]
          }
          frame "Start Recal" {
            n157 = RT FIFO Write(0:w467, 1:T14 {"Calibrated?"=FALSE, "IMU Detected?"=TRUE} ("element")) -> ()  [unwired: 3 in, 4 out]
            n158 = RT FIFO Write(0:w463, 1:T16 {"Command"=enum."Recalibrate", "Data"=0} ("element")) -> ()  [unwired: 3 in, 4 out]
          }
          frame "Configure Cal" {
            n159 = Bundle By Name(cluster=w473, "ADIS16448DevRef.Calibration Time"=w470) -> (w472:T13)
          }
        }
      }
    }
  }
  n160 = while {
    tunnel: w8 -> [w476]
    tunnel: [w475] -> w2
    stop <- w475 stop-if-true
    # "stop this VI when the VI calling StartComm goes idle"
    n161 = property class="VI"(reference=w476) -> ("Exec.State"=w478:T21)  [unwired: 1 in, 2 out]
    n162 = Wait (ms)(milliseconds to wait=u32 250) -> ()  [unwired: 1 out]
    n163 = Equal?(x=w478, y=T21."Idle" ("Execution:State")) -> (x = y?=w475:bool)
  }
  n164 = flat-sequence {
    tunnel: w2 -> [_]
    frame #0 {
      n165 = call <vilib>:"WPI_DigitalOutputRefNum Registry Get.vi"("refnum name"="448 Status LED") -> ("error out"=w485:errorcluster, "DigitalOutputDevRef"=w484:T17)  [unwired: 9 in]
      n166 = call <vilib>:"WPI_DigitalOutputClose.vi"("error in (no error)"=w485, "DigitalOutputDevRef"=w484) -> ("error out"=w480:errorcluster)  [unwired: 9 in]
      n167 = call <vilib>:"WPI_SPIRefNum Registry Get.vi"("error in (no error)"=w480, "refnum name"="AutoSPI") -> ("error out"=w482:errorcluster, "SPIDevRef"=w481:T12)  [unwired: 8 in]
      n168 = call <vilib>:"WPI_SPIClose.vi"("error in (no error)"=w482, "SPIDevRef"=w481) -> ()  [unwired: 9 in, 1 out]
    }
    frame #1 {
      n169 = Stop() -> ()  [unwired: 1 in]
    }
  }
